vi "main.vi"() -> ()   [LabVIEW 2019]
panel:
  out "lvl":string
  out "f":bool
  out "b":bool
  out "e":bool
  out "c":bool
  out "d":bool
  out "g":bool
  out "a":bool
  out "String 2":string
  out "1":bool
  out "3":bool
  out "2":bool
  out "border 4":bool
  out "border 3":bool
  out "border 2":bool
  out "border":bool
  in  "stop":bool
  out "WYNIK":i32
  out "Board":u32[][](array[colorbox])
  # "Astronauto witaj w grze Asteroids!\nTwoim celem jest zniszczenie wszystkich przeciwników\nw kosmosie na każdym z trzech poziomów. Liczy sie czas!\nZ każdą chwilą Twój wynik maleje, więc streszczaj sie!\n\nSTEROWANIE:\na/A - obracanie rakiety w prawo\nd/D - obracanie rakiety w lewy\nw/W - poruszanie sie w kierunku skierowania rakiety\nk/K - oddanie strzału"
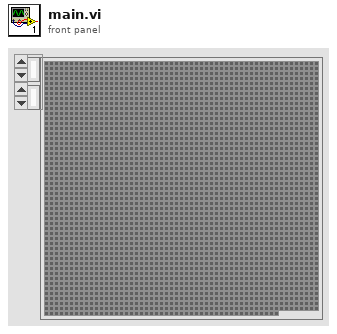
[diagram p1: front panel]
types:
  T1 = enum16{"skip", "prawo", "lewo", "ruch", "strzal"}
  T2 = cluster{u32[][], u32[][], u32[][], u32[][], u32[][], u32[][], u32[][], u32[][]}
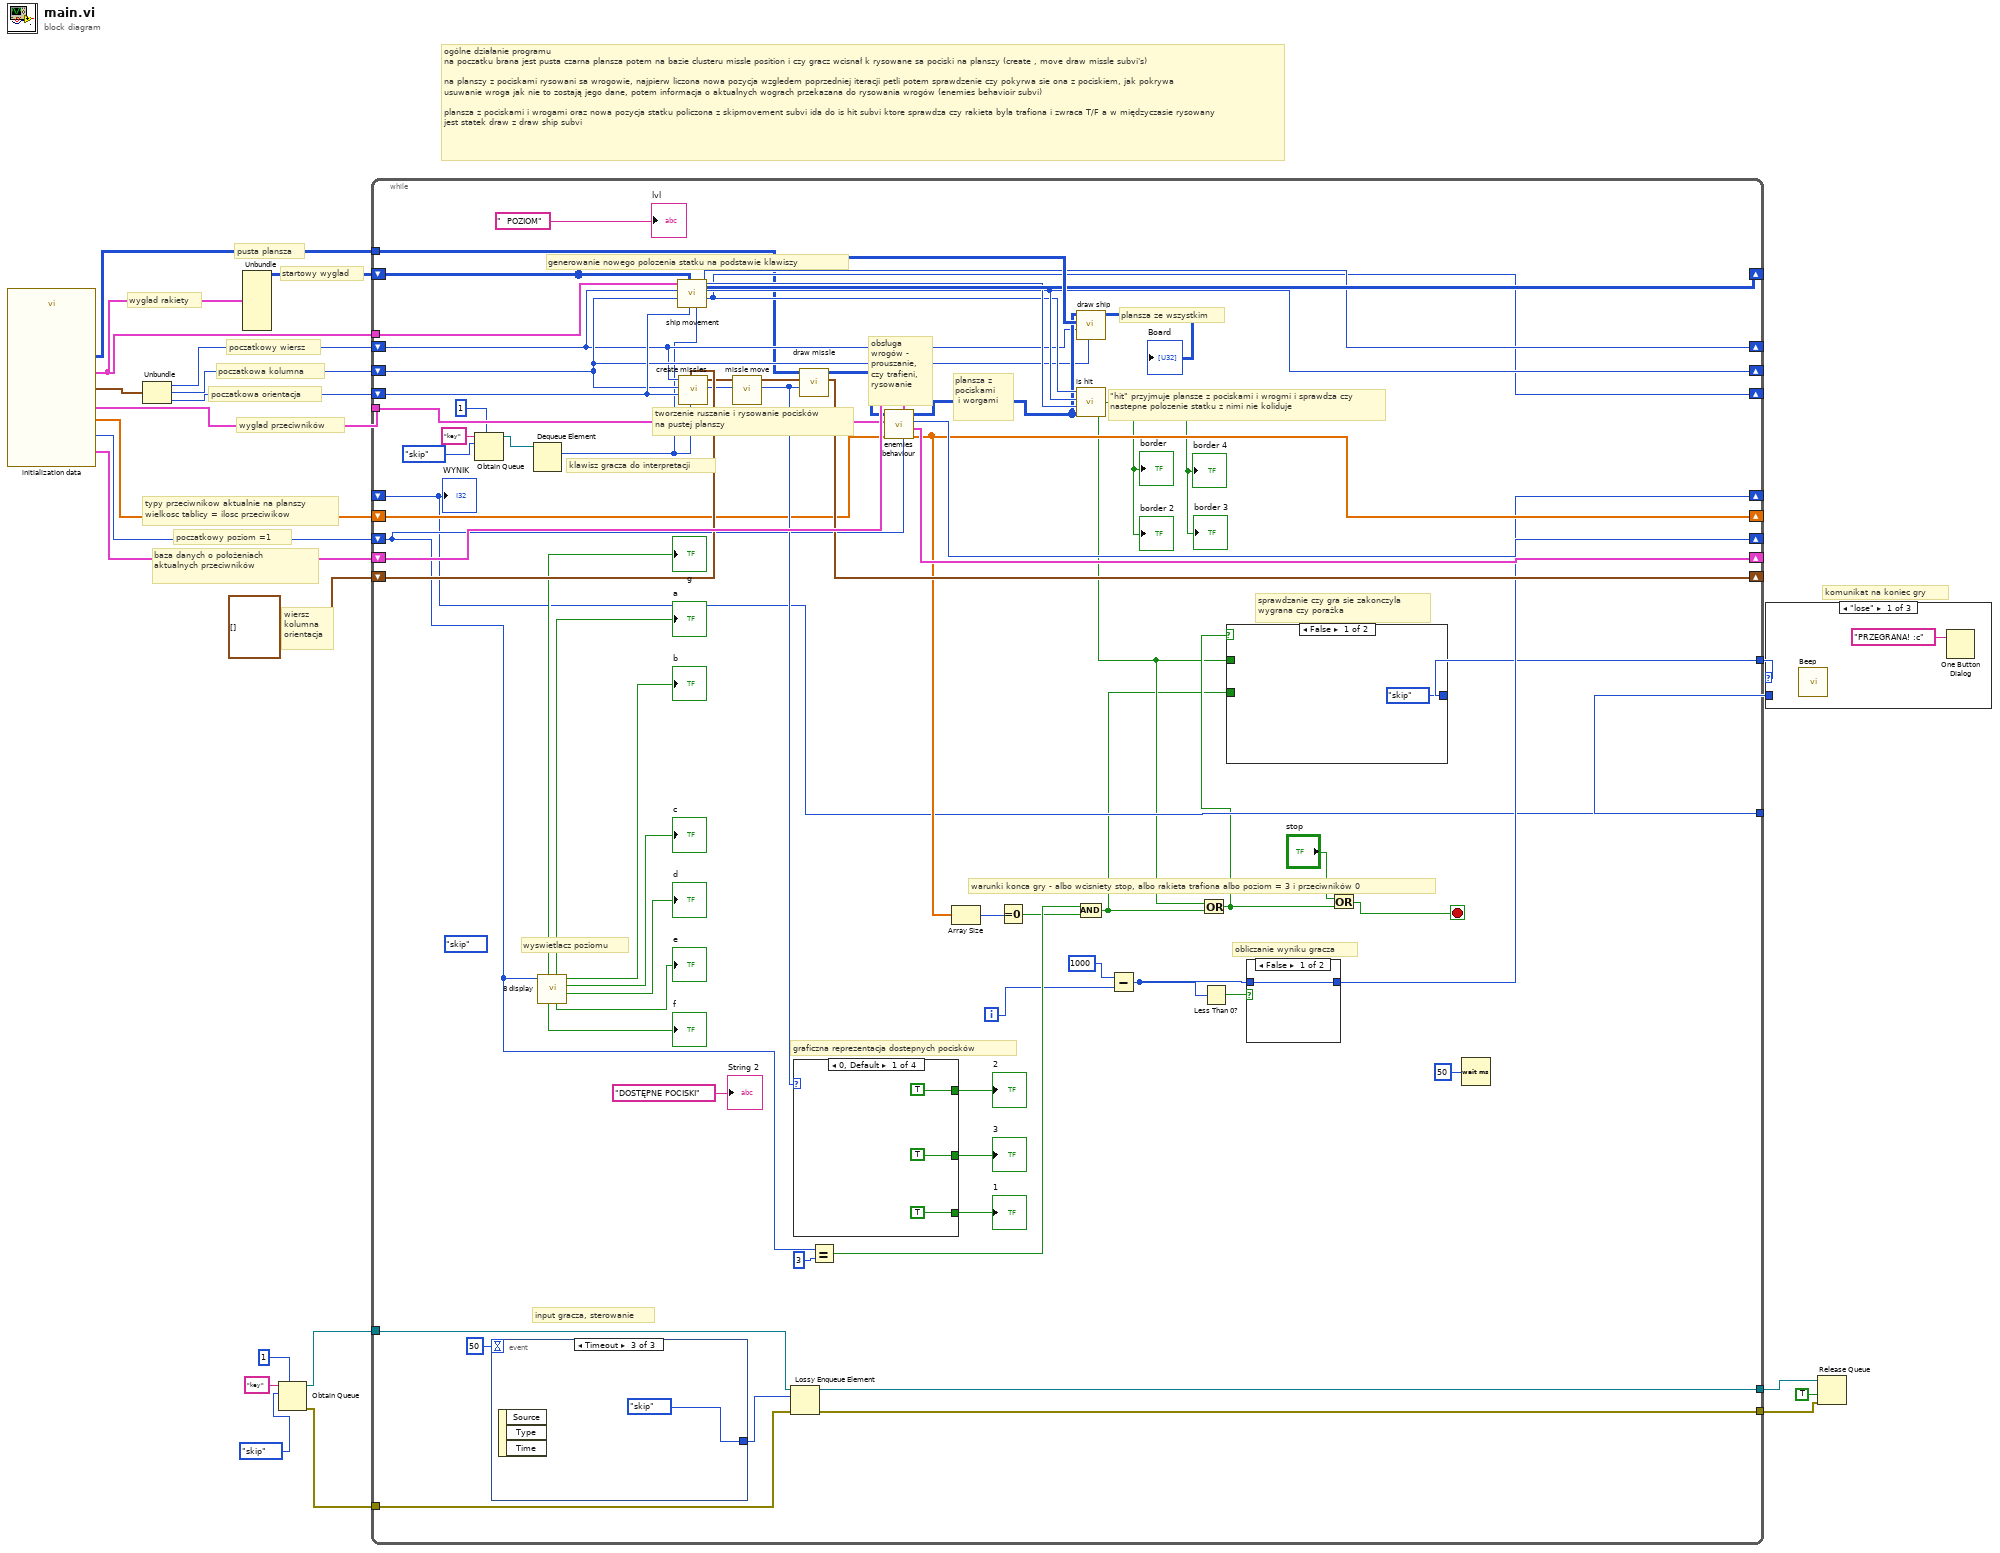
[diagram p0: block diagram]
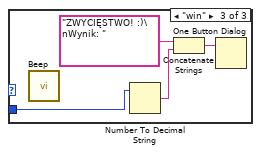
[diagram p3: hidden frame]
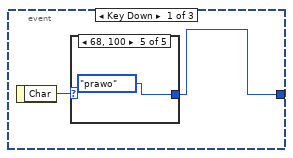
[diagram p4: hidden frame]
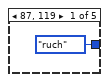
[diagram p5: hidden frame]
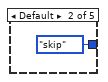
[diagram p6: hidden frame]
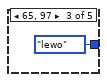
[diagram p7: hidden frame]
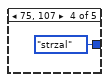
[diagram p8: hidden frame]
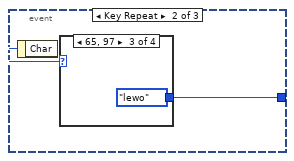
[diagram p9: hidden frame]
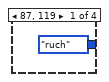
[diagram p10: hidden frame]
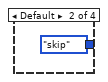
[diagram p11: hidden frame]
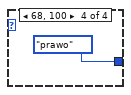
[diagram p12: hidden frame]
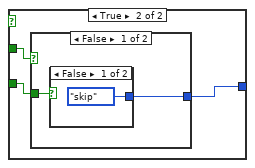
[diagram p13: hidden frame]
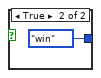
[diagram p14: hidden frame]
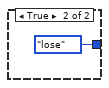
[diagram p15: hidden frame]
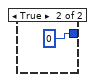
[diagram p16: hidden frame]
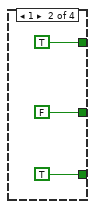
[diagram p17: hidden frame]
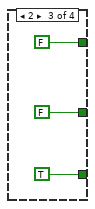
[diagram p18: hidden frame]
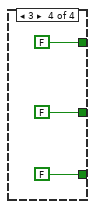
[diagram p19: hidden frame]
diagram:
  # "wiersz \nkolumna \norientacja"
  # "ogólne działanie programu\nna poczatku brana jest pusta czarna plansza potem na bazie clusteru missle position i czy gracz wcisnał k rysowane sa pociski na planszy (create , move draw missle subvi's)\n\nna planszy z pociskami rysowani sa wrogowie, najpierw liczona nowa pozycja wzgledem poprzedniej iteracji petli potem sprawdzenie czy pokyrwa sie ona z pociskiem, jak pokrywa usuwanie wroga jak nie to zostają jego dane, potem informacja o aktualnych wograch przekazana do rysowania wrogów (enemies behavioir subvi) \n\nplansza z pociskami i wrogami oraz nowa pozycja statku policzona z skipmovement subvi ida do is hit subvi ktore sprawdza czy rakieta byla trafiona i zwraca T/F a w międzyczasie rysowany jest statek draw z draw ship subvi"
  # "wyglad przeciwników"
  # "typy przeciwnikow aktualnie na planszy\nwielkosc tablicy = ilosc przeciwikow"
  # "baza danych o położeniach aktualnych przeciwników"
  # "poczatkowy poziom =1"
  # "komunikat na koniec gry"
  # "wyglad rakiety"
  # "pusta plansza"
  # "startowy wyglad"
  # "poczatkowa orientacja"
  # "poczatkowa kolumna"
  # "poczatkowy wiersz"
  n1 = call "initialization data.vi"() -> ("all enemies"=w15:cluster{u32[][], u32[][], u32[][], u32[][]}, "all ship orientations"=w20:T2, "ship initialozation coordiantes"=w19:cluster{i32, i32, i32}, "row column orientation every enemy initial"=w12:cluster{dbl[], dbl[], dbl[]}, "level"=w13:i32, "Board"=w22:u32[][], "enemies on board"=w14:dbl[])  [unwired: 4 in]
  n2 = Unbundle(w19) -> (w18:i32, w17:i32, w16:i32)
  n3 = Unbundle(w20) -> (w21:u32[][])  [unwired: 7 out]
  n4 = Obtain Queue(max queue size (-1, unlimited)=1, name (unnamed)="key", element data type=T1."skip") -> (queue out=w6:refnum<queue>, error out=w4:errorcluster)  [unwired: 2 in, 1 out]
  n5 = while {
    shift-right: [w83] -> _
    shift-left: w17 -> [w76]
    shift-right: [w84] -> _
    shift-left: w18 -> [w75]
    tunnel: w22 -> [w70]
    tunnel: w20 -> [w87]
    shift-right: [w85] -> _
    shift-left: w21 -> [w86]
    shift-right: [w82] -> _
    shift-left: w16 -> [w77]
    tunnel: w15 -> [w62]
    shift-right: [w47] -> _
    shift-left: w14 -> [w48]
    shift-right: [w61] -> _
    shift-left: w13 -> [w52]
    shift-right: [w78] -> _
    shift-left: w12 -> [w79]
    shift-right: [w68] -> _
    shift-left: cluster{i32, i32, i32}[] [] ("missles position out") -> [w74]
    shift-right: [w45] -> _
    shift-left: _ -> [w44]
    tunnel: [w44] -> w10
    tunnel: [w38] -> w9
    tunnel: w6 -> [w26]
    tunnel: w4 -> [w25]
    tunnel: [w24] -> w3
    tunnel: [w23] -> w2
    i -> [w35]
    stop <- w29 stop-if-true
    (unwired) T1."skip"
    # "klawisz gracza do interpretacji"
    # "warunki konca gry - albo wcisniety stop, albo rakieta trafiona albo poziom = 3 i przeciwników 0"
    # "graficzna reprezentacja dostepnych pocisków"
    # "wyswietlacz poziomu"
    # "generowanie nowego polozenia statku na podstawie klawiszy"
    # "obsługa wrogów - prouszanie,\nczy trafieni, rysowanie"
    # "tworzenie ruszanie i rysowanie pocisków\nna pustej planszy"
    # "\"hit\" przyjmuje plansze z pociskami i wrogmi i sprawdza czy nastepne polozenie statku z nimi nie koliduje"
    # "sprawdzanie czy gra sie zakonczyla \nwygrana czy porażka"
    # "input gracza, sterowanie"
    # "obliczanie wyniku gracza"
    # "plansza ze wszystkim"
    # "plansza z pociskami\n i worgami"
    n6 = Obtain Queue(max queue size (-1, unlimited)=1, name (unnamed)="key", element data type=T1."skip") -> (queue out=w33:refnum<queue>)  [unwired: 2 in, 2 out]
    n7 = event shown="[2] Timeout" {
      selector: _ -> [_ _ _]
      dyn-events: _ -> [_ _ _]
      timeout: 50 -> [_ _ _]
      tunnel: [w89 w96 T1."skip"] -> w27
      event Key Down {
        n8 = event-data() -> ("Char"=w90:i16)  [unwired: 1 in]
        n9 = case shown="68, 100" w90 {
          tunnel: [T1."ruch" enum16{"skip", "prawo", "lewo", "gora", "dol"}."skip" enum16{"skip", "prawo", "lewo", "gora", "dol"}."lewo" T1."strzal" enum16{"skip", "prawo", "lewo", "gora", "dol"}."prawo"] -> w89
          frame 87, 119 {
          }
          frame Default {
          }
          frame 65, 97 {
          }
          frame 75, 107 {
          }
          frame 68, 100 {
          }
        }
      }
      event Key Repeat {
        n10 = event-data() -> ("Char"=w97:i16)  [unwired: 1 in]
        n11 = case shown="65, 97" w97 {
          tunnel: [T1."ruch" enum16{"skip", "prawo", "lewo", "gora", "dol"}."skip" enum16{"skip", "prawo", "lewo", "gora", "dol"}."lewo" enum16{"skip", "prawo", "lewo", "gora", "dol"}."prawo"] -> w96
          frame 87, 119 {
          }
          frame Default {
          }
          frame 65, 97 {
          }
          frame 68, 100 {
          }
        }
      }
      event Timeout {
        n12 = event-data() -> ()  [unwired: 1 in, 3 out]
      }
    }
    n13 = Dequeue Element(queue=w33) -> (element=w34:T1)  [unwired: 2 in, 3 out]
    n14 = call "8 display.vi"("Numeric"=w52) -> ("d"=→"d":bool, "c"=→"c":bool, "b"=→"b":bool, "e"=→"e":bool, "a"=→"a":bool, "f"=→"f":bool, "g"=→"g":bool)  [unwired: 4 in]
    n15 = call "ship movement.vi"("key input"=w34, "orientation"=w77, "current position drawing"=w86, "column"=w76, "row"=w75, "all  position drawings"=w87) -> ("next orientation"=w82:i32, "next column"=w83:i32, "next row"=w84:i32, "next position drawing"=w85:u32[][])  [unwired: 2 in]
    n16 = call "create missles.vi"("key in"=w34, "current missles"=w74, "orinetation"=w77, "column"=w76, "row"=w75) -> ("number of missles"=w66:i32, "missles position out"=w67:cluster{i32, i32, i32}[])  [unwired: 5 in]
    n17 = call "missle move.vi"("number of missles"=w66, "missles position in"=w67) -> ("new number of missles"=w64:i32, "new missle position"=w65:cluster{i32, i32, i32}[])  [unwired: 8 in]
    n18 = Lossy Enqueue Element(queue=w26, element=w27, error in (no error)=w25) -> (queue out=w24:refnum<queue>, error out=w23:errorcluster)  [unwired: 2 out]
    n19 = case shown="0, Default" w64 {
      tunnel: [TRUE TRUE TRUE FALSE] -> w73
      tunnel: [TRUE TRUE FALSE FALSE] -> w72
      tunnel: [TRUE FALSE FALSE FALSE] -> w71
      frame 0, Default {
      }
      frame 1 {
      }
      frame 2 {
      }
      frame 3 {
      }
    }
    "2" <- w72
    "3" <- w71
    "1" <- w73
    n20 = call "draw missle.vi"("new number of missles"=w64, "new missle position in"=w65, "Board in"=w70) -> ("new missle position out"=w68:cluster{i32, i32, i32}[], "Board out"=w69:u32[][])  [unwired: 7 in]
    n21 = Equal?(x=w52, y=3) -> (x = y?=w50:bool)
    n22 = call "enemies behaviour.vi"("level"=w52, "row column orientation every enemy in"=w79, "enemies on board"=w48, "all enemies in"=w62, "Board with missles in"=w69) -> ("enemies on board out"=w47:dbl[], "row column orientation every enemy out"=w78:cluster{dbl[], dbl[], dbl[]}, "level out"=w61:i32, "Board with enemies"=w80:u32[][])  [unwired: 3 in]
    n23 = Array Size(array=w47) -> (size(s)=w37:i32)
    n24 = Equal To 0?(x=w37) -> (x = 0?=w49:bool)
    n25 = call "draw ship.vi"("column"=w76, "row"=w75, "ship position"=w86, "Board in"=w80) -> ("Board out"=→"Board":u32[][])  [unwired: 7 in]
    n26 = call "is hit.vi"("Board with rocks"=w80, "next row"=w84, "next column"=w83, "next orientation"=w82) -> ("is hit"=w40:bool)
    "border" <- w40
    "border 2" <- w40
    "border 3" <- w40
    "border 4" <- w40
    n27 = And(x=w50, y=w49) -> (x .and. y?=w39:bool)
    n28 = Subtract(x=1000, y=w35) -> (x-y=w36:i32)
    n29 = Or(x=w40, y=w39) -> (x .or. y?=w41:bool)
    n30 = Less Than 0?(x=w36) -> (x < 0?=w46:bool)
    n31 = case shown="False" w41 {
      tunnel: w40 -> [_ w106]
      tunnel: w39 -> [_ w105]
      tunnel: [enum16{"stop", "skip", "lose", "win"}."skip" w104] -> w38
      frame False {
      }
      frame True {
        n32 = case shown="False" w106 {
          tunnel: w105 -> [w108 _]
          tunnel: [w107 enum16{"stop", "skip", "lose", "win"}."lose"] -> w104
          frame False {
            n33 = case shown="False" w108 {
              tunnel: [enum16{"stop", "skip", "lose", "win"}."skip" enum16{"stop", "skip", "lose", "win"}."win"] -> w107
              frame False {
              }
              frame True {
              }
            }
          }
          frame True {
          }
        }
      }
    }
    n34 = case shown="False" w46 {
      tunnel: [w112 0 ("Score")] -> w45
      tunnel: w36 -> [w112 _]
      frame False {
      }
      frame True {
      }
    }
    n35 = Or(x="stop", y=w41) -> (x .or. y?=w29:bool)
    n36 = Wait (ms)(milliseconds to wait=u32 50) -> ()  [unwired: 1 out]
    "WYNIK" <- w44
    "String 2" <- "DOSTĘPNE POCISKI" ("String")
    "lvl" <- "  POZIOM" ("String 3")
  }
  n37 = case shown="\"lose\"" w9 {
    tunnel: w10 -> [_ _ w129]
    frame "lose" {
      n38 = call <vilib>:"Beep.vi"() -> ()  [unwired: 12 in]
      n39 = One Button Dialog(message="PRZEGRANA! :c") -> ()  [unwired: 1 in, 1 out]
    }
    frame "skip", Default {
    }
    frame "win" {
      n40 = call <vilib>:"Beep.vi"() -> ()  [unwired: 12 in]
      n41 = Number To Decimal String(number=w129) -> (decimal integer string=w128:string)  [unwired: 1 in]
      n42 = Concatenate Strings("ZWYCIĘSTWO! :)\nWynik: " ("message"), w128) -> (w127:string)
      n43 = One Button Dialog(message=w127) -> ()  [unwired: 1 in, 1 out]
    }
  }
  n44 = Release Queue(queue=w3, force destroy? (F)=TRUE, error in (no error)=w2) -> ()  [unwired: 3 out]
